vi "Set Message Type.vi"(8 "error in":errorcluster, 10 "message type":T1, 11 "message or subaddress":T2 format="%.0x") -> (0 "error out":errorcluster, 3 "message or subaddress out":T2 format="%.0x")   [LabVIEW 2020, in "AIM MIL-STD-1553 Scripting.lvlib"]
doc: "Sets the <b>message type</b> of the input <b>message or subaddress</b>."
uses:
  AIM MIL-STD-1553 Scripting.lvlib
  <vilib>/NI VeriStand/Custom Device API/Custom Device Item Ref.ctl
  Shared/Message Type.ctl
  Constants.vi
  <vilib>/NI VeriStand/Custom Device API/Set Item Property (String).vi
  <vilib>/NI VeriStand/Custom Device API/Custom Device API.lvlib
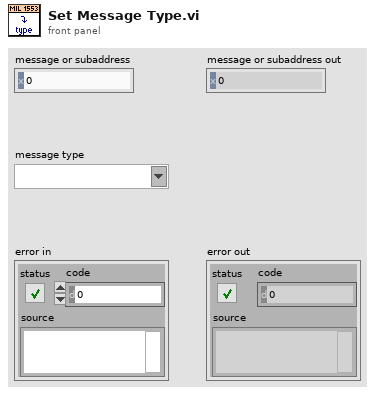
[diagram p1: front panel]
types:
  T1 = typedef "Message Type.ctl" = string
  T2 = typedef "Custom Device API.lvlib/Custom Device Item Ref.ctl" = u64
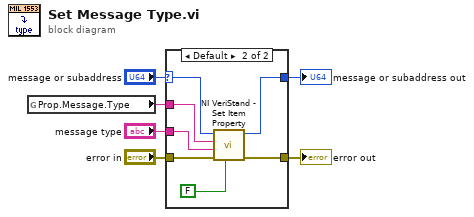
[diagram p0: block diagram]
diagram:
  n1 = global read "Constants.vi" "Prop.Message.Type"() -> (w2:string)
  n2 = case shown="Default" "message or subaddress" {
    selector: "message or subaddress" -> [w8 w15]
    tunnel: [w8 w14] -> w5
    tunnel: "error in" -> [w7 w13]
    tunnel: [w7 w12] -> w3
    tunnel: w2 -> [_ w11]
    tunnel: "message type" -> [_ w10]
    frame 0, -1 {
    }
    frame Default {
      n3 = call-poly <vilib>:"NI VeriStand - Set Item Property.vi"("Binary String (T)"=FALSE, "error in (no error)"=w13, "Value"=w10, "Property Name"=w11, "Item Ref in"=w15) -> ("error out"=w12:errorcluster, "Item Ref out"=w14:T2)  [unwired: 4 in, 1 out]
    }
  }
  "message or subaddress out" <- w5
  "error out" <- w3
